vi "NNF_Top_PXI(8Cores).vi"() -> ()   [LabVIEW 2020]
uses:
  <vilib>/Ngene/DeepLTK FPGA Addon/Toolkit/NNF_FPGA/Low_Level/Controls/NNCE_Controls.ctl
  <vilib>/Ngene/DeepLTK FPGA Addon/Toolkit/DeepLTK_FPGA_Addon.lvlib
  <vilib>/rvi/DataTransferAndStorage/Container/XNode/niFpgaContainer.xnode
  <vilib>/rvi/DataTransferAndStorage/Register/Emulation/niFpgaRegisterEmulationRefIn.vi
  <vilib>/rvi/LocalResourceManager/LocalResourceManager.xnode
  <vilib>/rvi/eio/common/nirviEmuReportErrorAndStop.vi
  <vilib>/rvi/DataTransferAndStorage/Container/Common/niFpgaContainerGetUniqueNameForEmu.vi
  <vilib>/rvi/DataTransferAndStorage/Container/Common/niFpgaContainerSetEmuInfo.vi
  <vilib>/Ngene/DeepLTK FPGA Addon/Toolkit/NNF_FPGA/Low_Level/Controls/Resource_Ref_Cfg/NNCE_Resource_Ref_Cfg_8ch.ctl
  <vilib>/Ngene/DeepLTK FPGA Addon/Toolkit/NNF_Host/Low_Level/NNF_Init/Controls/NNF_FPGA_Target_Info.ctl
  <vilib>/rvi/FIFO/Fifo_Resource/niFpgaFifoEmulationRefIn.vi
  <vilib>/Ngene/DeepLTK FPGA Addon/Toolkit/NNF_FPGA/API/Host_Shared_Controls/NNCE_Network_CFG.ctl
  <vilib>/Ngene/DeepLTK FPGA Addon/Toolkit/NNF_FPGA/API/Host_Shared_Controls/Memory_Selecter.ctl
  <vilib>/Ngene/DeepLTK FPGA Addon/Toolkit/NNF_FPGA/API/Host_Shared_Controls/NNCE_Activation_Type.ctl
  <vilib>/Ngene/DeepLTK FPGA Addon/Toolkit/NNF_FPGA/API/Host_Shared_Controls/Pulling_type.ctl
  <vilib>/Ngene/DeepLTK FPGA Addon/Toolkit/NNF_FPGA/API/Host_Shared_Controls/NNCE_Layer_CFG.ctl
panel:
  in  "NNF_Config":T1={"L"=0, "Layers"=[{"Pad ?"=FALSE, "W"=0.0, "H"=0.0, "CB"=0.0, "KB"=0.0, "Source"=enum."DMA", "Dest"=enum."DMA", "Activation"=enum."Sigmoid", "Pool_type"=enum."Avg", "BI_Offset"=0.0}, {"Pad ?"=FALSE, "W"=0.0, "H"=0.0, "CB"=0.0, "KB"=0.0, "Source"=enum."DMA", "Dest"=enum."DMA", "Activation"=enum."Sigmoid", "Pool_type"=enum."Avg", "BI_Offset"=0.0}, {"Pad ?"=FALSE, "W"=0.0, "H"=0.0, "CB"=0.0, "KB"=0.0, "Source"=enum."DMA", "Dest"=enum."DMA", "Activation"=enum."Sigmoid", "Pool_type"=enum."Avg", "BI_Offset"=0.0}, {"Pad ?"=FALSE, "W"=0.0, "H"=0.0, "CB"=0.0, "KB"=0.0, "Source"=enum."DMA", "Dest"=enum."DMA", "Activation"=enum."Sigmoid", "Pool_type"=enum."Avg", "BI_Offset"=0.0}, {"Pad ?"=FALSE, "W"=0.0, "H"=0.0, "CB"=0.0, "KB"=0.0, "Source"=enum."DMA", "Dest"=enum."DMA", "Activation"=enum."Sigmoid", "Pool_type"=enum."Avg", "BI_Offset"=0.0}, {"Pad ?"=FALSE, "W"=0.0, "H"=0.0, "CB"=0.0, "KB"=0.0, "Source"=enum."DMA", "Dest"=enum."DMA", "Activation"=enum."Sigmoid", "Pool_type"=enum."Avg", "BI_Offset"=0.0}, {"Pad ?"=FALSE, "W"=0.0, "H"=0.0, "CB"=0.0, "KB"=0.0, "Source"=enum."DMA", "Dest"=enum."DMA", "Activation"=enum."Sigmoid", "Pool_type"=enum."Avg", "BI_Offset"=0.0}, {"Pad ?"=FALSE, "W"=0.0, "H"=0.0, "CB"=0.0, "KB"=0.0, "Source"=enum."DMA", "Dest"=enum."DMA", "Activation"=enum."Sigmoid", "Pool_type"=enum."Avg", "BI_Offset"=0.0}, {"Pad ?"=FALSE, "W"=0.0, "H"=0.0, "CB"=0.0, "KB"=0.0, "Source"=enum."DMA", "Dest"=enum."DMA", "Activation"=enum."Sigmoid", "Pool_type"=enum."Avg", "BI_Offset"=0.0}, {"Pad ?"=FALSE, "W"=0.0, "H"=0.0, "CB"=0.0, "KB"=0.0, "Source"=enum."DMA", "Dest"=enum."DMA", "Activation"=enum."Sigmoid", "Pool_type"=enum."Avg", "BI_Offset"=0.0}, {"Pad ?"=FALSE, "W"=0.0, "H"=0.0, "CB"=0.0, "KB"=0.0, "Source"=enum."DMA", "Dest"=enum."DMA", "Activation"=enum."Sigmoid", "Pool_type"=enum."Avg", "BI_Offset"=0.0}, {"Pad ?"=FALSE, "W"=0.0, "H"=0.0, "CB"=0.0, "KB"=0.0, "Source"=enum."DMA", "Dest"=enum."DMA", "Activation"=enum."Sigmoid", "Pool_type"=enum."Avg", "BI_Offset"=0.0}, {"Pad ?"=FALSE, "W"=0.0, "H"=0.0, "CB"=0.0, "KB"=0.0, "Source"=enum."DMA", "Dest"=enum."DMA", "Activation"=enum."Sigmoid", "Pool_type"=enum."Avg", "BI_Offset"=0.0}, {"Pad ?"=FALSE, "W"=0.0, "H"=0.0, "CB"=0.0, "KB"=0.0, "Source"=enum."DMA", "Dest"=enum."DMA", "Activation"=enum."Sigmoid", "Pool_type"=enum."Avg", "BI_Offset"=0.0}, {"Pad ?"=FALSE, "W"=0.0, "H"=0.0, "CB"=0.0, "KB"=0.0, "Source"=enum."DMA", "Dest"=enum."DMA", "Activation"=enum."Sigmoid", "Pool_type"=enum."Avg", "BI_Offset"=0.0}, {"Pad ?"=FALSE, "W"=0.0, "H"=0.0, "CB"=0.0, "KB"=0.0, "Source"=enum."DMA", "Dest"=enum."DMA", "Activation"=enum."Sigmoid", "Pool_type"=enum."Avg", "BI_Offset"=0.0}], "Relative Scale"=[0.0, 0.0, 0.0, 0.0, 0.0, 0.0, 0.0, 0.0, 0.0, 0.0, 0.0, 0.0, 0.0, 0.0, 0.0, 0.0, 0.0, 0.0, 0.0, 0.0, 0.0, 0.0, 0.0, 0.0, 0.0, 0.0, 0.0, 0.0, 0.0, 0.0, 0.0, 0.0], "Bias Scale"=[0.0, 0.0, 0.0, 0.0, 0.0, 0.0, 0.0, 0.0, 0.0, 0.0, 0.0, 0.0, 0.0, 0.0, 0.0, 0.0, 0.0, 0.0, 0.0, 0.0, 0.0, 0.0, 0.0, 0.0, 0.0, 0.0, 0.0, 0.0, 0.0, 0.0, 0.0, 0.0]}
  in  "Run":bool
  out "Exec_Iter":i32
  in  "Init":bool
  in  "Flush timer":i16
  in  "Total Channels":u16
  out "Target Information":T6
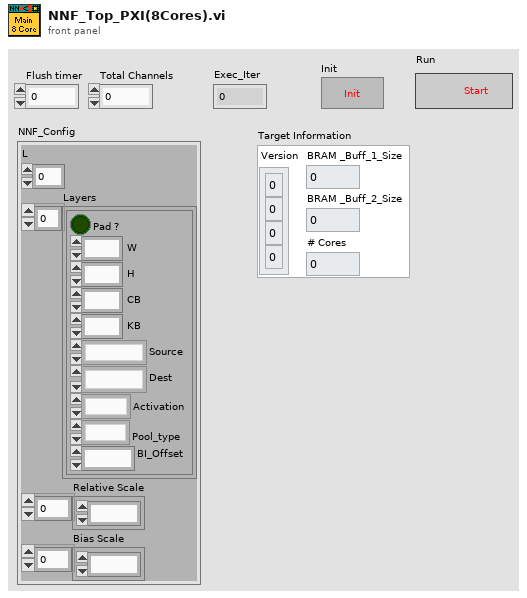
[diagram p1: front panel]
types:
  T1 = typedef "DeepLTK_FPGA_Addon.lvlib/NNCE_Network_CFG.ctl" = cluster{"L":u8, "Layers":T2[], "Relative Scale":fxp<+,16,5>[], "Bias Scale":fxp<+,16,5>[]}
  T2 = typedef "DeepLTK_FPGA_Addon.lvlib/NNCE_Layer_CFG.ctl" = cluster{"Pad ?":bool, "W":fxp<+,9,9>, "H":fxp<+,9,9>, "CB":fxp<+,10,10>, "KB":fxp<+,10,10>, "Source":T3, "Dest":T3, "Activation":T4, "Pool_type":T5, "BI_Offset":fxp<+,12,12>}
  T3 = typedef "DeepLTK_FPGA_Addon.lvlib/Memory_Selecter.ctl" = enum8{"DMA", "BRAM1", "BRAM2"}
  T4 = typedef "DeepLTK_FPGA_Addon.lvlib/NNCE_Activation_Type.ctl" = enum8{"Sigmoid", "ReLU", "LReLU", "MaxOut", "tanh", "None"}
  T5 = typedef "DeepLTK_FPGA_Addon.lvlib/Pulling_type.ctl" = enum8{"None", "Max", "Avg"}
  T6 = typedef "DeepLTK_FPGA_Addon.lvlib/NNF_FPGA_Target_Info.ctl" = cluster{"BRAM _Buff_1_Size":u32, "BRAM _Buff_2_Size":u32, "Version":u8[], "# Cores":u32}
  T7 = typedef "DeepLTK_FPGA_Addon.lvlib/NNCE_Resource_Ref_Cfg_8ch.ctl" = cluster{"Engine_Clock":refnum<k21>, "DMA_Data_In":refnum<k21>, "DMA_Data_Out":refnum<k21>, "DMA_Weights_In":refnum<k21>, "DMA_Bias_K_Scalers_In":refnum<k21>, "BRAM_Buff_1":refnum<k21>, "BRAM_Buff_2":refnum<k21>}
  T8 = typedef "DeepLTK_FPGA_Addon.lvlib/NNCE_Controls.ctl" = cluster{"Flush timer ":i16, "Total_Channels":u16}
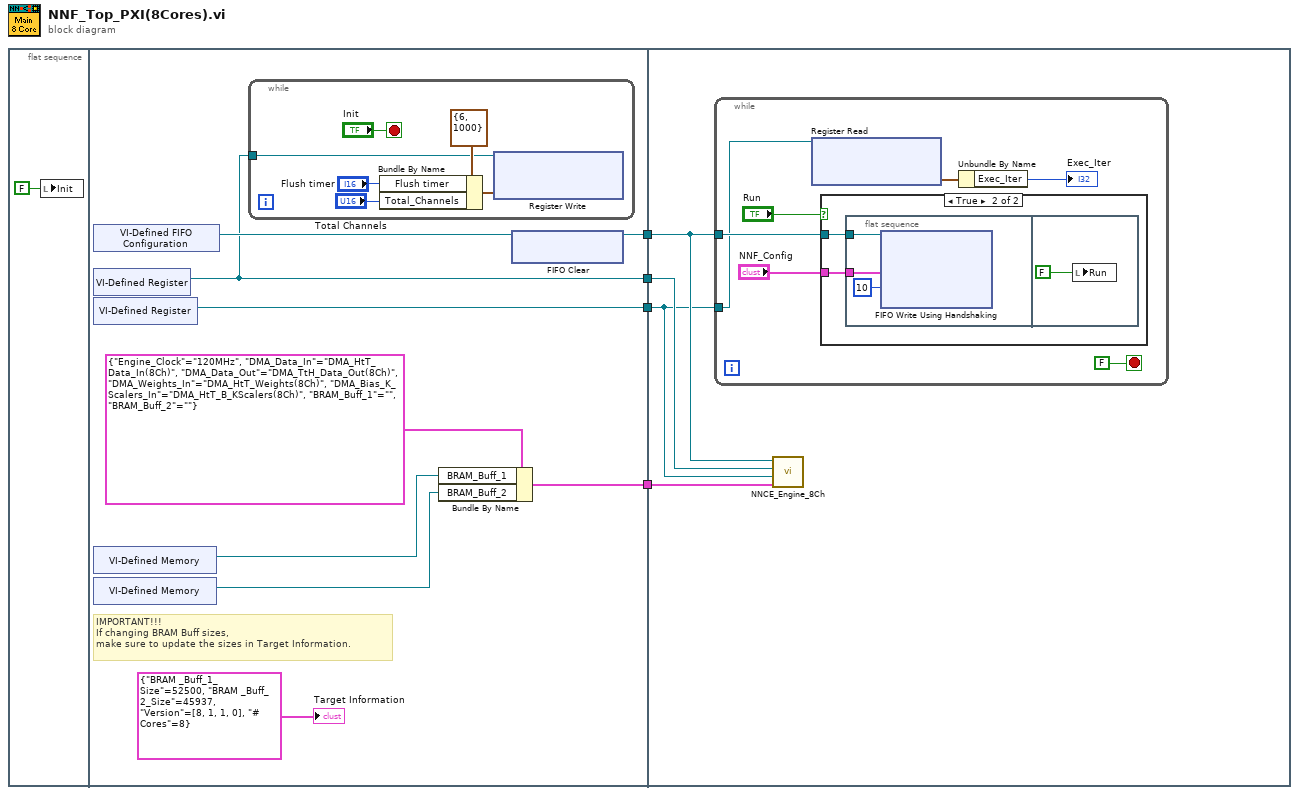
[diagram p0: block diagram]
diagram:
  n1 = flat-sequence {
    tunnel: [w6] -> w4
    tunnel: [w13] -> w3
    tunnel: [w8] -> w2
    tunnel: [w7] -> w1
    tunnel: w4 -> [w24]
    tunnel: w3 -> [w23]
    tunnel: w2 -> [w22]
    tunnel: w1 -> [w21]
    frame #0 {
      n2 = local write "Init"(FALSE ("Start")) -> ()
    }
    frame #1 {
      # "IMPORTANT!!!\nIf changing BRAM Buff sizes,\nmake sure to update the sizes in Target Information."
      n3 = xnode "VI-Defined FIFO Configuration"() -> ("FIFO Out"=w11:refnum<k21>)
      n4 = xnode "VI-Defined Register"() -> ("Register Out"=w8:refnum<k21>)
      n5 = xnode "VI-Defined Register"() -> ("Register Out"=w7:refnum<k21>)
      n6 = xnode "VI-Defined Memory"() -> ("Memory Out"=w12:refnum<k21>)
      n7 = xnode "VI-Defined Memory"() -> ("Memory Out"=w9:refnum<k21>)
      n8 = while {
        tunnel: w8 -> [w16]
        stop <- "Init" stop-if-true
        n9 = Bundle By Name(cluster=T8 {"Flush timer "=6, "Total_Channels"=1000} ("Cluster"), "Flush timer"="Flush timer", "Total_Channels"="Total Channels") -> (w15:T8)
        n10 = xnode ("Register Write")("Data"=w15, "Register In"=w16) -> ()  [unwired: 1 out]
      }
      n11 = Bundle By Name(cluster=T7 {"Engine_Clock"="120MHz", "DMA_Data_In"="DMA_HtT_Data_In(8Ch)", "DMA_Data_Out"="DMA_TtH_Data_Out(8Ch)", "DMA_Weights_In"="DMA_HtT_Weights(8Ch)", "DMA_Bias_K_Scalers_In"="DMA_HtT_B_KScalers(8Ch)", "BRAM_Buff_1"="", "BRAM_Buff_2"=""} ("NNCE_Resource_Cfg"), "BRAM_Buff_1"=w12, "BRAM_Buff_2"=w9) -> (w13:T7)
      n12 = xnode ("FIFO Clear")("FIFO In"=w11) -> ("FIFO Out"=w6:refnum<k21>)
      "Target Information" <- T6 {"BRAM _Buff_1_Size"=52500, "BRAM _Buff_2_Size"=45937, "Version"=[8, 1, 1, 0], "# Cores"=8} ("Cluster")
    }
    frame #2 {
      n13 = while {
        tunnel: w24 -> [w31]
        tunnel: w21 -> [w27]
        stop <- FALSE stop-if-true
        n14 = xnode ("Register Read")("Register In"=w27) -> ("Data"=w26:cluster{"Exec_Iter":i32})  [unwired: 1 out]
        n15 = case shown="True" "Run" {
          tunnel: w31 -> [_ w33]
          tunnel: "NNF_Config" -> [_ w32]
          frame False {
          }
          frame True {
            n16 = flat-sequence {
              tunnel: w33 -> [w36]
              tunnel: w32 -> [w35]
              frame #0 {
                n17 = xnode ("FIFO Write Using Handshaking")("Element"=w35, "Timeout"=10, "FIFO In"=w36) -> ()  [unwired: 2 out]
              }
              frame #1 {
                n18 = local write "Run"(FALSE ("Start")) -> ()
              }
            }
          }
        }
        n19 = Unbundle By Name(w26) -> ("Exec_Iter"=→"Exec_Iter":i32)
      }
      n20 = call <vilib>:"NNCE_Engine_8Ch.vi"("NNCE_Resource_Cfg"=w23, "NNCE_Indicators"=w21, "NNCE_Controls"=w22, "Configuration FIFO"=w24) -> ()  [unwired: 8 in]
    }
  }
